vi "Set Pre Trigger Percent.vi"(8 "error in (no error)":errorcluster, 11 "front":i32) -> (0 "error out":errorcluster)   [LabVIEW 2023, in "vmmsolib.lvlib"]
doc: "DLL_API void WINAPI SetPreTriggerPercent(int front);"
uses:
  vmmsolib.lvlib
  vmmso.dll
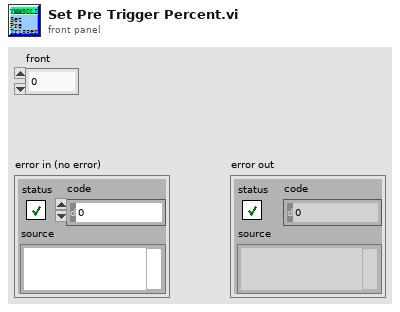
[diagram p1: front panel]
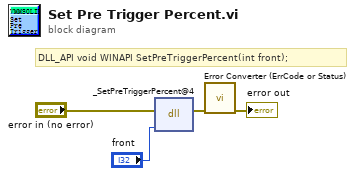
[diagram p0: block diagram]
diagram:
  # "DLL_API void WINAPI SetPreTriggerPercent(int front);"
  n1 = dll-call lib="D:/VmMsoSDK/demo-Labview/2023/vmmsolib/vmmso.*" fn="_SetPreTriggerPercent@4"(error in="error in (no error)", "front"="front") -> (error out=w2:errorcluster)  [unwired: 4 in, 1 out]
  n2 = call "Error Converter (ErrCode or Status).vi"("error in (no error)"=w2) -> ("error out"=→"error out":errorcluster)  [unwired: 10 in]
